vi "Create Enhanced Config JSON.vi"(11 "Value":variant) -> (0 "error out":errorcluster, 3 "PAtools JSON":string)   [LabVIEW 2023]
uses:
  Plugin/AMS Climate Chamber Template/Configuration Params.ctl
  <vilib>/ADAS Replay HIL/Template Node/Plugin/Template Node/Common Configuration Params.ctl
  Capabilities/Capabilities/High Level Capabilities/Climate Chamber Cluster/Climate Chamber Cluster.lvclass
  Capabilities/Capabilities/Utilities/Utilities.lvlib
  <vilib>/ADAS Replay HIL/AdasCommonUtilities/AdasCommonUtilities.lvlib
  <vilib>/ADAS Replay HIL/Template Node/Plugin/Template Node/Template Node.lvclass
  Plugin/AMS Climate Chamber Template/AMS Climate Chamber Template.lvclass
panel:
  in  "Custom Parameters":T1={"Common"={"Iteration Interval (s)"=0.001, "T0 (ns)"=0, "Priority"=100, "Processor"=-2, "Wait in Ready State"=TRUE}, "Amount of Channels"=1, "Address"=""} {"Common"."Iteration Interval (s)" format="%#_13g"}
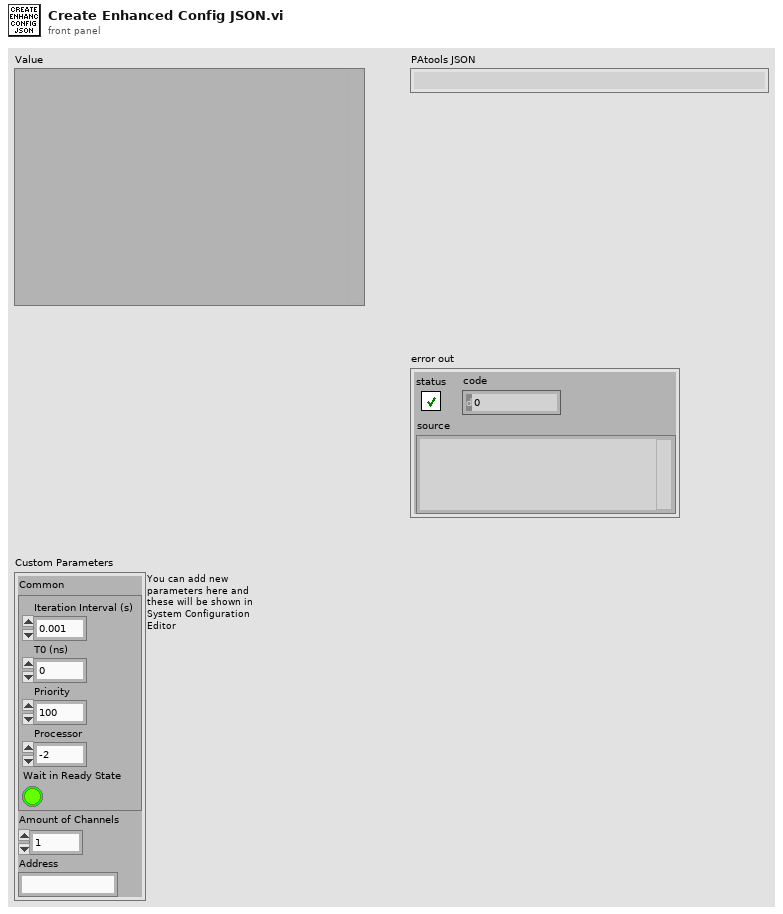
[diagram p1: front panel]
types:
  T1 = typedef "AMS Climate Chamber Template.lvlib/AMS Climate Chamber Template.lvclass/Configuration Params.ctl" = cluster{"Common":T2, "Amount of Channels":u32, "Address":string}
  T2 = typedef "Template Node.lvlib/Template Node.lvclass/Common Configuration Params.ctl" = cluster{"Iteration Interval (s)":dbl, "T0 (ns)":u64, "Priority":i32, "Processor":i32, "Wait in Ready State":bool}
  T3 = typedef "NI_App_Builder_API.lvlib/Build Specification Version.ctl" = cluster{"Major":u16, "Minor":u16, "Fix":u16, "Build":u16}
  T4 = typedef "Utilities.lvlib/Channel.ctl" = cluster{"Title":string, "SubTitle":string[], "Consumer?":bool, "Name":string, "Description":string, "Size":i32, "OffSets":i32[], "DataType":string[], "DefaultValue":dbl[]}
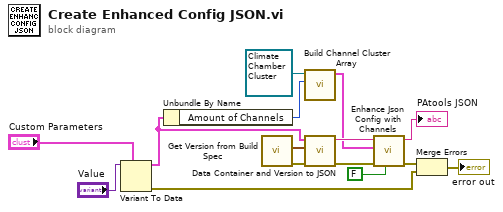
[diagram p0: block diagram]
diagram:
  n1 = Variant To Data(type="Custom Parameters", Variant="Value") -> (data=w10:T1, error out=w7:errorcluster)  [unwired: 1 in]
  n2 = Unbundle By Name(w10) -> ("Amount of Channels"=w2:u32)
  n3 = call "Get Version from Build Spec.vi"() -> ("error out"=w8:errorcluster, "Version"=w15:T3)  [unwired: 8 in, 2 out]
  n4 = call-dynamic "Build Channel Cluster Array.vi"("Climate Chamber Cluster.lvclass in"=refnum<class "Climate Chamber Cluster.lvclass"> refnum ("Climate Chamber Cluster.lvclass"), "Channels Amount"=w2) -> ("Channels out"=w3:cluster{"Channels":T4[]})  [unwired: 8 in]
  n5 = call <vilib>:"Data Container and Version to JSON.vi"("error in (no error)"=w8, "Version"=w15, "Container Variant"=w10) -> ("error out"=w12:errorcluster, "JSON string"=w14:string)  [unwired: 7 in]
  n6 = call "Enhance Json Config with Channels.vi"("Save PAtools config Json? (Default: True)"=FALSE ("Save PAtools config Json?"), "error in"=w12, "Channels"=w3, "Json Config"=w14) -> ("error out"=w6:errorcluster, "PAtools JSON"=→"PAtools JSON":string)  [unwired: 6 in]
  n7 = Merge Errors(w6, w7) -> (→"error out":errorcluster)
